vi "DIO64 Load.vi"(0 "board in":u16 format="%.0x", 1 "input hint":i32=-1, 2 "output hint":i32=-1, 5 "filename":path, 11 "error in (no error)":errorcluster) -> (4 "board out":u16 format="%.0x", 15 "error out":errorcluster)   [LabVIEW 2012]
doc: "DIO64 Load loads the designated FPGA code onto the DIO-64 board.\n\nCopyright (c) 2002 Viewpoint Systems Inc. All Rights Reserved"
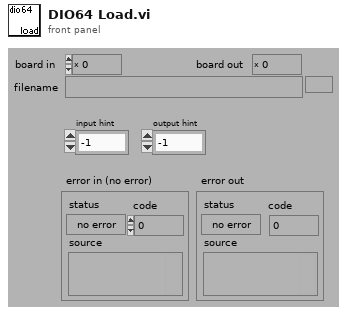
[diagram p1: front panel]
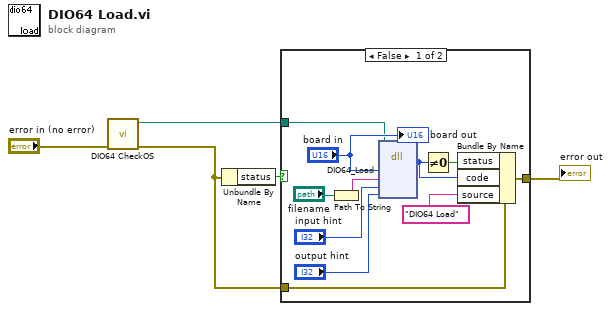
[diagram p0: block diagram]
diagram:
  n1 = call "DIO64 CheckOS.vi"("error in"="error in (no error)") -> ("error out"=w1:errorcluster, "path in"=w3:path)  [unwired: 9 in]
  n2 = Unbundle By Name(w1) -> ("status"=w5:bool)
  n3 = case shown="False" w5 {
    tunnel: w1 -> [w13 w17]
    tunnel: [w12 w17] -> w4
    tunnel: w3 -> [w6 _]
    frame False {
      n4 = Path To String(path="filename") -> (string=w10:string)
      n5 = dll-call lib="C:/DIO64Visa/DLL/DIO64_Visa32/Debug/DIO64_Visa32.dll" fn="DIO64_Load"(path in=w6, "board"="board in", "filename"=w10, "ihint"="input hint", "ohint"="output hint") -> ("return type"=w16:i32)  [unwired: 6 in, 2 out]
      n6 = Not Equal To 0?(x=w16) -> (x != 0?=w15:bool)
      n7 = Bundle By Name(cluster=w13, "status"=w15, "code"=w16, "source"="DIO64 Load") -> (w12:errorcluster)
      "board out" <- "board in"
    }
    frame True {
    }
  }
  "error out" <- w4
